vi "InitRGBStudentVersion.vi"(2 "error in (no error)":errorcluster) -> ()   [LabVIEW 2019]
uses:
  <vilib>/myRIO/Instrument Drivers/Onboard IO/I2C/typedefs/I2C Transfer Rate.ctl
  <vilib>/myRIO/Instrument Drivers/Onboard IO/I2C/I2C.lvlib
  <vilib>/myRIO/Instrument Drivers/Onboard IO/I2C/typedefs/I2C User Configuration.ctl
  <vilib>/myRIO/Instrument Drivers/Onboard IO/I2C/typedefs/I2C Configuration.ctl
  <vilib>/myRIO/Common/Instrument Driver Framework/myRIO v1.0/I2C/typedefs/I2C Channels Enum.ctl
  <vilib>/myRIO/Common/Instrument Driver Framework/Utilities/typedefs/Generic FPGA Reference.ctl
  <vilib>/myRIO/Common/Instrument Driver Framework/Utilities/typedefs/myRIO v1.0 Reference.ctl
  <vilib>/myRIO/Common/Instrument Driver Framework/Utilities/typedefs/Hardware Version Enum.ctl
  <vilib>/myRIO/Common/Instrument Driver Framework/Utilities/typedefs/myRIO Generic Hardware Reference.ctl
  <vilib>/myRIO/Instrument Drivers/Onboard IO/I2C/typedefs/I2C Reference.ctl
  <vilib>/myRIO/Instrument Drivers/Onboard IO/I2C/vis/Configure.vi
  <vilib>/myRIO/Instrument Drivers/Onboard IO/I2C/vis/Write Read.vi
  <vilib>/userDefined/High Color/nirio_resource_hc.ctl
  <vilib>/myRIO/Common/Instrument Driver Framework/myRIO v1.0/I2C/vis/myRIO v1.1 Open I2C.vi
  <vilib>/myRIO/Instrument Drivers/Onboard IO/I2C/vis/myRIO I2C Open.xnode
  <vilib>/myRIO/Common/Instrument Driver Framework/Utilities/vis/Is FPGA Ref Available.vi
  <vilib>/myRIO/Express VI/Onboard IO/I2C/I2C Express VI.xnode
panel:
  in  "stop":bool
  in  "High":string="—"
  in  "Low":string="–"
  out "Total":u32
  out "error out 2":errorcluster
  out "Low 2":u8[](array[numeric])
  out "High 2":u8[](array[numeric])
  # "RED: 22 23"
  # "GREEN: 24 25"
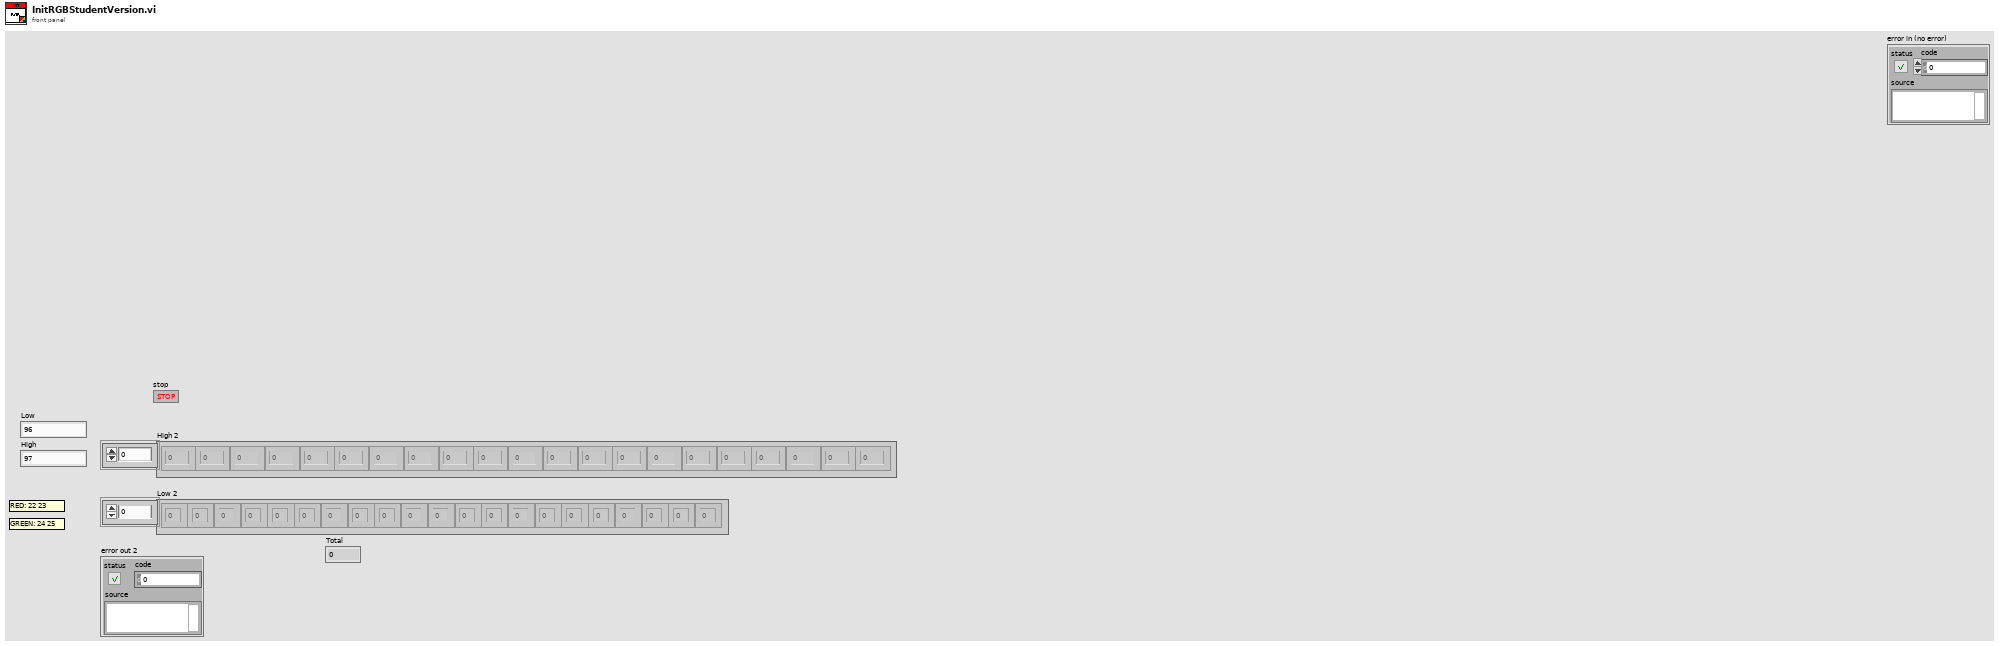
[diagram p1: front panel]
types:
  T1 = typedef "I2C.lvlib/I2C Reference.ctl" = cluster{"myRIO Reference":T2, "I2C Channels Enum":T6, "I2C Configuration":T7}
  T2 = typedef "myRIO Generic Hardware Reference.ctl" = cluster{"myRIO Model":T3, "myRIO Hardware Reference":T4}
  T3 = typedef "Hardware Version Enum.ctl" = enum16{"Unknown", "myRIO-1900", "myRIO-1950", "roboRIO", "NI ELVIS RIO CM", "ELVIS III"}
  T4 = typedef "myRIO v1.0 Reference.ctl" = cluster{"Generic FPGA Reference":T5, "Allow multiple opens":bool}
  T5 = typedef "Generic FPGA Reference.ctl" = refnum<k20>
  T6 = typedef "I2C Channels Enum.ctl" = enum16{"Not Connected", "A/I2C", "B/I2C", "I2C/I2C"}
  T7 = typedef "I2C.lvlib/I2C Configuration.ctl" = cluster{"I2C Transfer Rate":T8}
  T8 = typedef "I2C.lvlib/I2C Transfer Rate.ctl" = enum16{"Standard mode (100 kbps)", "Fast mode (400 kbps)"}
  T9 = typedef "I2C.lvlib/I2C User Configuration.ctl" = cluster{"I2C Transfer Rate":T8}
  T10 = typedef "nirio_resource_hc.ctl" = tag
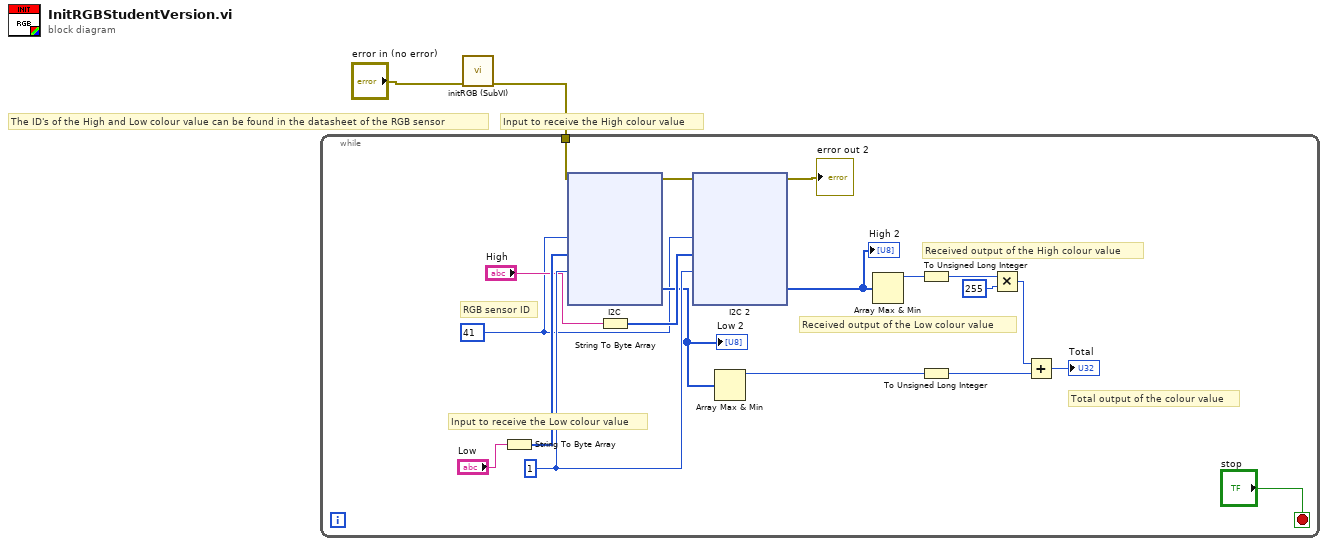
[diagram p0: block diagram]
diagram:
  # "The ID's of the High and Low colour value can be found in the datasheet of the RGB sensor"
  # "Input to receive the High colour value"
  n1 = call "initRGB (SubVI).vi"("error in (no error)"="error in (no error)") -> ("error out"=w1:errorcluster)  [unwired: 10 in]
  n2 = while {
    tunnel: w1 -> [w3]
    stop <- "stop" stop-if-true
    w5 = 41 ("Numeric")
    w18 = u32 1 ("Byte Count")
    # "Total output of the colour value"
    # "Received output of the Low colour value"
    # "Received output of the High colour value"
    # "Input to receive the Low colour value"
    # "RGB sensor ID"
    n3 = String To Byte Array(string="Low") -> (unsigned byte array=w17:u8[])
    n4 = xnode "I2C"("Slave Address (7-bit)"=w5, "Bytes to Write"=w17, "Byte Count"=w18, "error in (no error)"=w3) -> ("Bytes Read"=w14:u8[], "error out"=w19:errorcluster)
    "Low 2" <- w14
    n5 = String To Byte Array(string="High") -> (unsigned byte array=w16:u8[])
    n6 = xnode "I2C 2"("Slave Address (7-bit)"=w5, "Bytes to Write"=w16, "Byte Count"=w18, "error in (no error)"=w19) -> ("Bytes Read"=w13:u8[], "error out"=→"error out 2":errorcluster)
    "High 2" <- w13
    n7 = Array Max & Min(array=w14) -> (max value=w7:u8)  [unwired: 3 out]
    n8 = Array Max & Min(array=w13) -> (max value=w9:u8)  [unwired: 3 out]
    n9 = To Unsigned Long Integer(number=w9) -> (unsigned 32bit integer=w8:u32)
    n10 = To Unsigned Long Integer(number=w7) -> (unsigned 32bit integer=w6:u32)
    n11 = Multiply(x=w8, y=u32 255) -> (x*y=w11:u32)
    n12 = Add(x=w11, y=w6) -> (x+y=→"Total":u32)
  }
